vi "Get Log File Properties.vi"(8 "error in (no error)":errorcluster, 10 "System Channel Refnums":T2[](array[typedef]) format="%.0x", 11 "Device Reference in":T2 format="%.0x") -> (0 "error out":errorcluster, 2 "Log File Properties":T1)   [LabVIEW 2019, in "Telemetry Engine.lvlib"]
uses:
  Telemetry Engine.lvlib
  <vilib>/NI VeriStand/Custom Device API/Custom Device Item Ref.ctl
  Types/Log File Properties.ctl
  <vilib>/NI VeriStand/Custom Device API/Custom Device API.lvlib
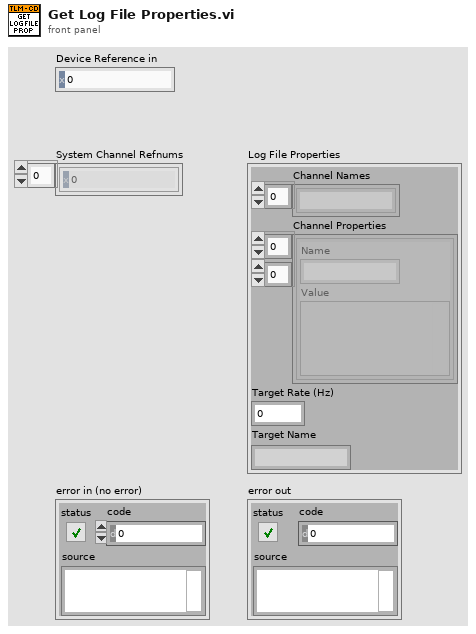
[diagram p1: front panel]
types:
  T1 = typedef "Telemetry Engine.lvlib/Log File Properties.ctl" = cluster{"Channel Names":string[], "Channel Properties":cluster{"Name":string, "Value":variant}[][], "Target Rate (Hz)":dbl, "Target Name":string}
  T2 = typedef "Custom Device API.lvlib/Custom Device Item Ref.ctl" = u64
  T3 = typedef "Custom Device API.lvlib/Custom Device Item Info.ctl" = cluster{"Name":string, "Is Channel":bool, "GUID":string, "Is Waveform":bool}
  T4 = cluster{"Description":string, "Variant":variant}[]
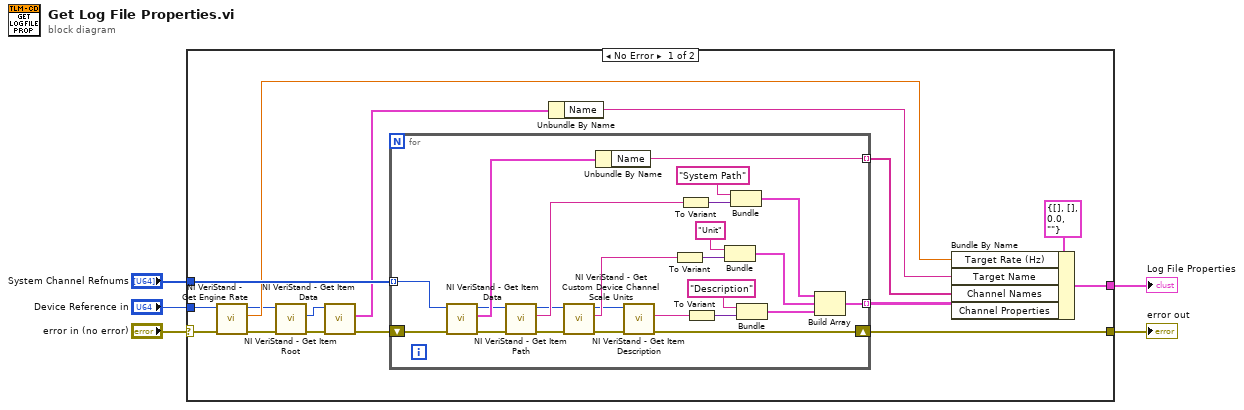
[diagram p0: block diagram]
diagram:
  n1 = case shown="No Error" "error in (no error)" {
    selector: "error in (no error)" -> [w19 w46]
    tunnel: "Device Reference in" -> [w13 _]
    tunnel: [w21 w46] -> w4
    tunnel: "System Channel Refnums" -> [w20 _]
    tunnel: [w15 _] -> w1
    frame No Error {
      n2 = call <vilib>:"NI VeriStand - Get Engine Rate.vi"("error in (no error)"=w19, "Item Ref in"=w13) -> ("error out"=w11:errorcluster, "Rate (Hz)"=w14:dbl, "Item Ref out"=w10:T2)  [unwired: 7 in]
      n3 = call <vilib>:"NI VeriStand - Get Item Root.vi"("error in (no error)"=w11, "Item Ref in"=w10) -> ("error out"=w12:errorcluster, "Root Ref out"=w9:T2)  [unwired: 6 in, 2 out]
      n4 = call <vilib>:"NI VeriStand - Get Item Data.vi"("error in (no error)"=w12, "Item Ref in"=w9) -> ("error out"=w7:errorcluster, "Item Info"=w8:T3)  [unwired: 6 in, 2 out]
      n5 = for {
        tunnel: w20 -> [w44] mode=indexing
        shift-right: [w43] -> w21
        shift-left: w7 -> [w32]
        tunnel: [w42] -> w16 mode=indexing
        tunnel: [w22] -> w18 mode=indexing
        n6 = call <vilib>:"NI VeriStand - Get Item Data.vi"("error in (no error)"=w32, "Item Ref in"=w44) -> ("error out"=w37:errorcluster, "Item Info"=w45:T3, "Item Ref out"=w31:T2)  [unwired: 6 in, 1 out]
        n7 = call <vilib>:"NI VeriStand - Get Item Path.vi"("error in (no error)"=w37, "Item Ref in"=w31) -> ("error out"=w30:errorcluster, "Path"=w34:string, "Item Ref out"=w28:T2)  [unwired: 6 in, 1 out]
        n8 = call <vilib>:"NI VeriStand - Get Custom Device Channel Scale Units.vi"("error in (no error)"=w30, "Channel Ref in"=w28) -> ("error out"=w29:errorcluster, "ScaleUnits"=w25:string, "Channel Ref out"=w24:T2)  [unwired: 7 in]
        n9 = Unbundle By Name(w45) -> ("Name"=w42:string)
        n10 = call <vilib>:"NI VeriStand - Get Item Description.vi"("error in (no error)"=w29, "Item Ref in"=w24) -> ("error out"=w43:errorcluster, "Description"=w41:string)  [unwired: 6 in, 2 out]
        n11 = To Variant(anything=w25) -> (Variant=w27:variant)
        n12 = To Variant(anything=w34) -> (Variant=w35:variant)
        n13 = To Variant(anything=w41) -> (Variant=w40:variant)
        n14 = Bundle("Description"="Unit", "Variant"=w27) -> (w23:cluster{"Description":string, "Variant":variant})  [unwired: 1 in]
        n15 = Bundle("Description"="System Path", "Variant"=w35) -> (w33:cluster{"Description":string, "Variant":variant})  [unwired: 1 in]
        n16 = Bundle("Description"="Description", "Variant"=w40) -> (w38:cluster{"Description":string, "Variant":variant})  [unwired: 1 in]
        n17 = Build Array(w33, w23, w38) -> (w22:T4)
      }
      n18 = Unbundle By Name(w8) -> ("Name"=w6:string)
      n19 = Bundle By Name(cluster=T1 {"Channel Names"=[], "Channel Properties"=[], "Target Rate (Hz)"=0.0, "Target Name"=""} ("input cluster"), "Target Rate (Hz)"=w14, "Target Name"=w6, "Channel Names"=w16, "Channel Properties"=w18) -> (w15:T1)
    }
    frame Error {
    }
  }
  "error out" <- w4
  "Log File Properties" <- w1
